vi "Service-Panel.vi"() -> ()   [LabVIEW 2021]
uses:
  Global-Var-OperService.vi
  Global-Var-Simulator.vi
panel:
  in  "service_work_end_btn":bool
  in  "service_work_start_btn":bool
  in  "service_call_got_btn":bool
  out "service_work_in_progress_ind":bool
  out "service_new_call_ind":bool
  in  "carWash2_alarms_list_btn":bool
  in  "carWash1_alarms_list_btn":bool
  out "carWash_2_alarm_ind_2":bool
  out "carWash_1_alarm_ind_2":bool
  in  "shiner_filled_btn":bool
  in  "soap_filled_btn":bool
  in  "water_filled_btn":bool
  out "shiner_level_ind":dbl
  out "soap_level_ind":dbl
  out "water_level_ind":dbl
  out "shiner_level_tank":dbl(slide) scale=0.0..500.0
  out "soap_level_tank":dbl(slide) scale=0.0..500.0
  out "water_level_tank":dbl(slide) scale=0.0..500.0
  in  "home_btn":bool
  # "Alarmy"
  # "Myjnia Południe"
  # "Myjnia Północ"
  # "Poziomy płynów w zbiornikach"
  # "Zgłoszenie"
  # "Nowe zgłoszenie"
  # "Woda"
  # "Mydło"
  # "Nabłyszczacz"
  # "Praca w toku"
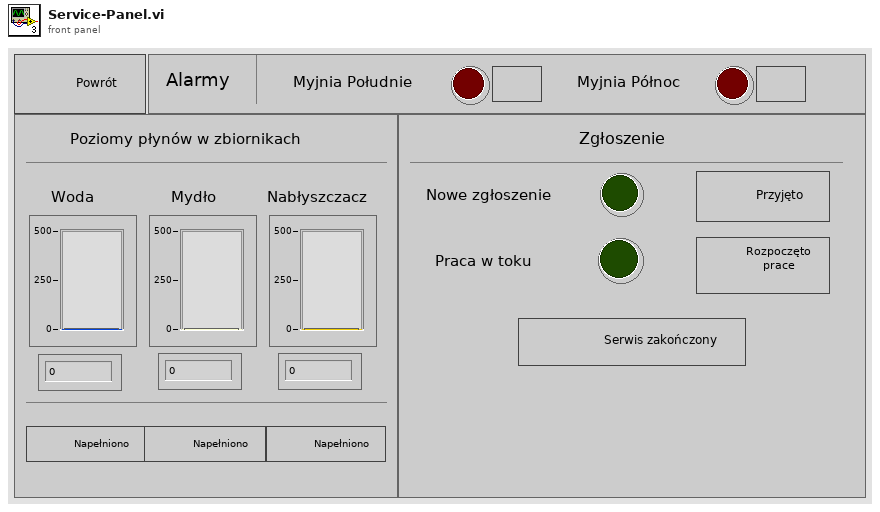
[diagram p1: front panel]
types:
  T1 = enum32{"Invalid", "Standard", "Closed", "Hidden", "Minimized", "Maximized"}
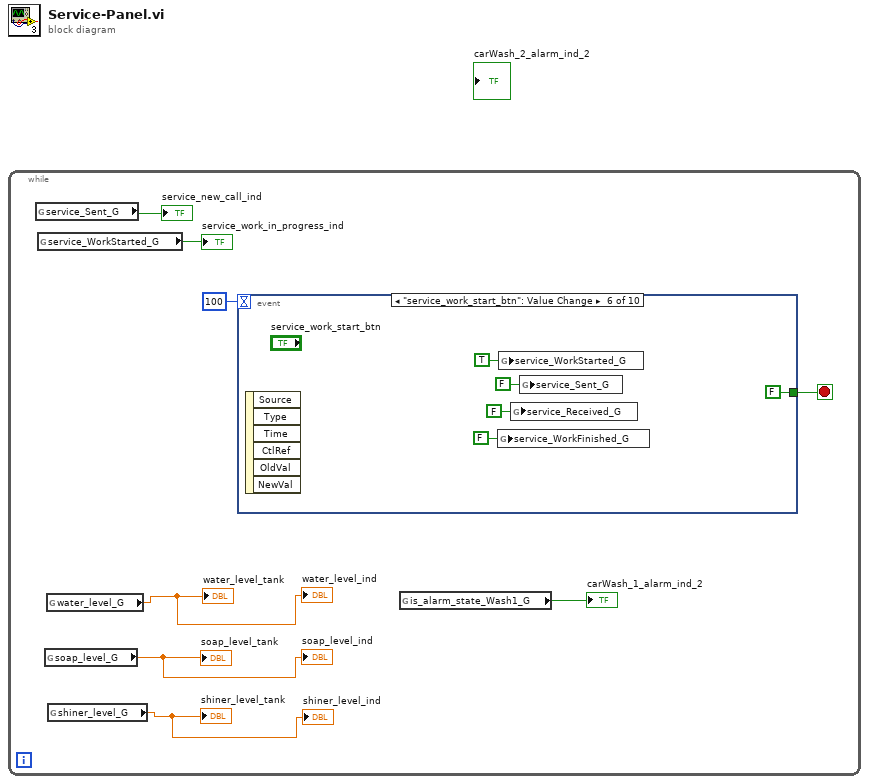
[diagram p0: block diagram]
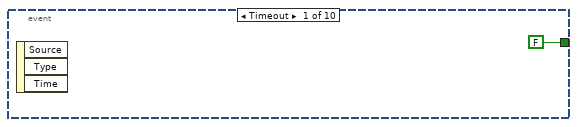
[diagram p2: hidden frame]
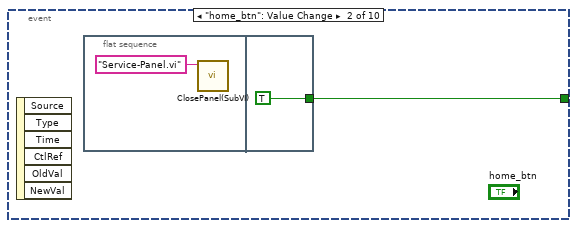
[diagram p3: hidden frame]
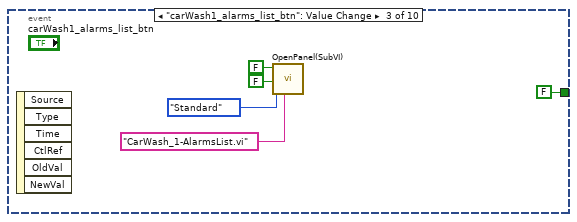
[diagram p4: hidden frame]
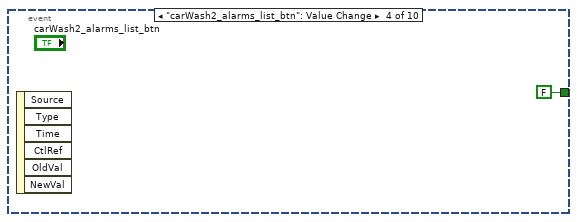
[diagram p5: hidden frame]
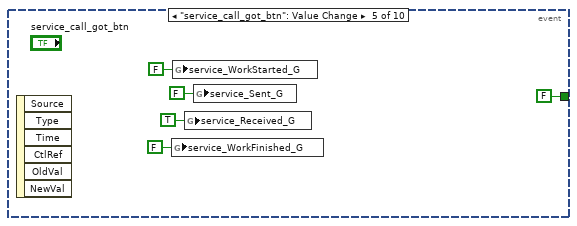
[diagram p6: hidden frame]
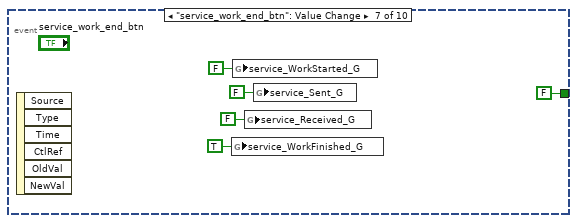
[diagram p7: hidden frame]
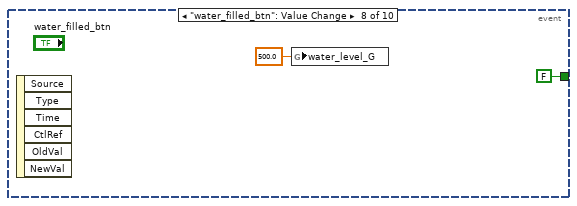
[diagram p8: hidden frame]
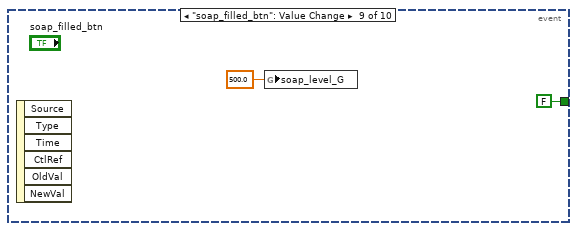
[diagram p9: hidden frame]
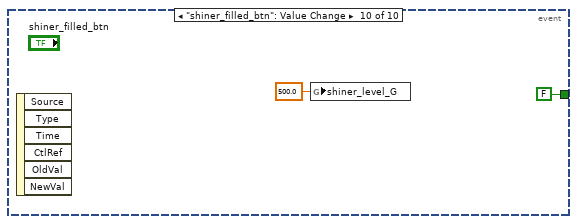
[diagram p10: hidden frame]
diagram:
  n1 = while {
    stop <- w7 stop-if-true
    n2 = global read "Global-Var-OperService.vi" "service_Sent_G"() -> (→"service_new_call_ind":bool)
    n3 = global read "Global-Var-OperService.vi" "service_WorkStarted_G"() -> (→"service_work_in_progress_ind":bool)
    n4 = global read "Global-Var-Simulator.vi" "soap_level_G"() -> (→"soap_level_tank" →"soap_level_ind":dbl)
    n5 = global read "Global-Var-Simulator.vi" "water_level_G"() -> (→"water_level_tank" →"water_level_ind":dbl)
    n6 = global read "Global-Var-Simulator.vi" "shiner_level_G"() -> (→"shiner_level_tank" →"shiner_level_ind":dbl)
    n7 = event shown="[5] \"service_work_start_btn\": Value Change" {
      selector: _ -> [_ _ _ _ _ _ _ _ _ _]
      dyn-events: _ -> [_ _ _ _ _ _ _ _ _ _]
      timeout: 100 -> [_ _ _ _ _ _ _ _ _ _]
      tunnel: [FALSE w10 FALSE FALSE FALSE FALSE FALSE FALSE FALSE FALSE] -> w7
      event Timeout {
        n8 = event-data() -> ()  [unwired: 1 in, 3 out]
      }
      event "home_btn": Value Change {
        n9 = event-data() -> ()  [unwired: 1 in, 6 out]
        n10 = flat-sequence {
          tunnel: [TRUE] -> w10
          frame #0 {
            n11 = call "ClosePanel(SubVI).vi"("String"="Service-Panel.vi") -> ()  [unwired: 11 in]
          }
          frame #1 {
          }
        }
      }
      event "carWash1_alarms_list_btn": Value Change {
        n12 = event-data() -> ()  [unwired: 1 in, 6 out]
        n13 = call "OpenPanel(SubVI).vi"("String"="CarWash_1-AlarmsList.vi", "State"=T1."Standard", "Wait Until Done"=FALSE, "Auto Dispose Reference"=FALSE) -> ()  [unwired: 8 in]
      }
      event "carWash2_alarms_list_btn": Value Change {
        n14 = event-data() -> ()  [unwired: 1 in, 6 out]
      }
      event "service_call_got_btn": Value Change {
        n15 = event-data() -> ()  [unwired: 1 in, 6 out]
        n16 = global write "Global-Var-OperService.vi" "service_WorkFinished_G"(FALSE ("service_WorkFinished_G")) -> ()
        n17 = global write "Global-Var-OperService.vi" "service_WorkStarted_G"(FALSE ("service_WorkStarted_G")) -> ()
        n18 = global write "Global-Var-OperService.vi" "service_Received_G"(TRUE ("service_Received_G")) -> ()
        n19 = global write "Global-Var-OperService.vi" "service_Sent_G"(FALSE ("service_Sent_G")) -> ()
      }
      event "service_work_start_btn": Value Change {
        n20 = event-data() -> ()  [unwired: 1 in, 6 out]
        n21 = global write "Global-Var-OperService.vi" "service_WorkFinished_G"(FALSE ("service_WorkFinished_G")) -> ()
        n22 = global write "Global-Var-OperService.vi" "service_WorkStarted_G"(TRUE ("service_WorkStarted_G")) -> ()
        n23 = global write "Global-Var-OperService.vi" "service_Received_G"(FALSE ("service_Received_G")) -> ()
        n24 = global write "Global-Var-OperService.vi" "service_Sent_G"(FALSE ("service_Sent_G")) -> ()
      }
      event "service_work_end_btn": Value Change {
        n25 = event-data() -> ()  [unwired: 1 in, 6 out]
        n26 = global write "Global-Var-OperService.vi" "service_WorkFinished_G"(TRUE ("service_WorkFinished_G")) -> ()
        n27 = global write "Global-Var-OperService.vi" "service_WorkStarted_G"(FALSE ("service_WorkStarted_G")) -> ()
        n28 = global write "Global-Var-OperService.vi" "service_Received_G"(FALSE ("service_Received_G")) -> ()
        n29 = global write "Global-Var-OperService.vi" "service_Sent_G"(FALSE ("service_Sent_G")) -> ()
      }
      event "water_filled_btn": Value Change {
        n30 = event-data() -> ()  [unwired: 1 in, 6 out]
        n31 = global write "Global-Var-Simulator.vi" "water_level_G"(500.0 ("water_level_G")) -> ()
      }
      event "soap_filled_btn": Value Change {
        n32 = event-data() -> ()  [unwired: 1 in, 6 out]
        n33 = global write "Global-Var-Simulator.vi" "soap_level_G"(500.0 ("water_level_G")) -> ()
      }
      event "shiner_filled_btn": Value Change {
        n34 = event-data() -> ()  [unwired: 1 in, 6 out]
        n35 = global write "Global-Var-Simulator.vi" "shiner_level_G"(500.0 ("water_level_G")) -> ()
      }
    }
    n36 = global read "Global-Var-Simulator.vi" "is_alarm_state_Wash1_G"() -> (→"carWash_1_alarm_ind_2":bool)
  }
